vi "TestWriteBlk2.vi"() -> ()   [LabVIEW 2011]
panel:
  out "添加的数组":string[][](array[string])
  out "Image Pixels (U8)":u8[][][][](array[numeric])
  out "数值":i32
  out "偏移量（字节） 2":i64
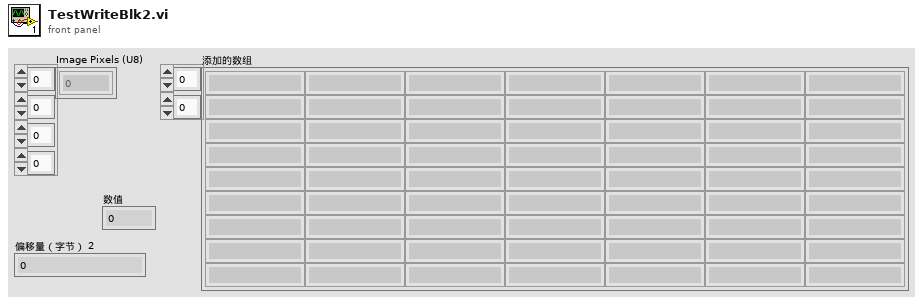
[diagram p1: front panel]
types:
  T1 = enum16{"big-endian, network order", "native, host order", "little-endian"}
  T2 = typedef "IMAQ Image.ctl" = refnum<image>
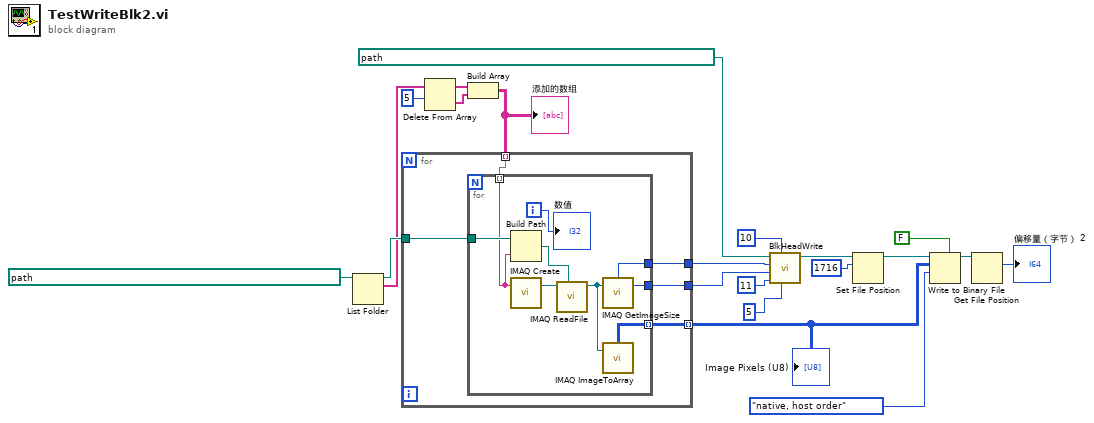
[diagram p0: block diagram]
diagram:
  n1 = List Folder(path=path "C:/Documents and Settings/pan/桌面/热成像/testimaging" ("路径")) -> (path out=w19:path, filenames=w5:string[])  [unwired: 3 in, 2 out]
  n2 = Delete From Array(array=w5, length=5 ("长度")) -> (deleted portion=w2:string[], array with subset deleted=w3:string[])  [unwired: 1 in]
  n3 = Build Array(w3, w2) -> (w1:string[][])
  "添加的数组" <- w1
  n4 = for {
    tunnel: w19 -> [w26]
    tunnel: [w25] -> w18
    tunnel: [w24] -> w17
    tunnel: [w23] -> w13 mode=indexing
    tunnel: w1 -> [w22] mode=indexing
    n5 = for {
      tunnel: w26 -> [w35]
      tunnel: [w32] -> w23 mode=indexing
      tunnel: [w30] -> w25
      tunnel: [w29] -> w24
      tunnel: w22 -> [w27] mode=indexing
      i -> [w28]
      n6 = Build Path(base path=w35, name or relative path=w27) -> (appended path=w34:path)
      n7 = call "IMAQ Create"("Image Name"=w27) -> ("New Image"=w33:T2)  [unwired: 4 in, 1 out]
      n8 = call "IMAQ ReadFile"("File Path"=w34, "Image"=w33) -> ("Image Out"=w31:T2)  [unwired: 5 in, 4 out]
      n9 = call "IMAQ GetImageSize"("Image"=w31) -> ("Y Resolution"=w29:i32, "X Resolution"=w30:i32)  [unwired: 3 in, 1 out]
      n10 = call "IMAQ ImageToArray"("Image"=w31) -> ("Image Pixels (U8)"=w32:u8[][])  [unwired: 3 in, 4 out]
      "数值" <- w28
    }
  }
  "Image Pixels (U8)" <- w13
  n11 = call "BlkHeadWrite.vi"("Stimuli"=5, "FramesPerStim"=10, "datatype"=11, "FrameHeight"=w17, "FrameWidth"=w18, "BlkFilePath"=path "C:/Documents and Settings/pan/桌面/热成像/WriteTest4D.blk") -> ("引用句柄输出"=w8:refnum<file>)  [unwired: 5 in]
  n12 = Set File Position(offset (in bytes) (0)=i64 1716 ("偏移量（字节）（0）"), refnum=w8) -> (refnum out=w9:refnum<file>)  [unwired: 2 in, 1 out]
  n13 = Write to Binary File(file (use dialog)=w9, data=w13, 5:FALSE ("预置数组或字符串大小？(T)"), 9:T1."native, host order" ("字节顺序(0:big-endian, network order)")) -> (refnum out=w12:refnum<file>)  [unwired: 2 in, 2 out]
  n14 = Get File Position(7:w12) -> (2:→"偏移量（字节） 2":i64)  [unwired: 1 in, 2 out]
